vi "Changed Mode.vi"(8 "error in (no error)":errorcluster, 11 "Instrument in":refnum<class "Instrument.lvclass">) -> (0 "error out":errorcluster, 3 "Instrument out":refnum<class "Instrument.lvclass">)   [LabVIEW 2018, in "Instrument.lvclass"]
uses:
  Instrument.lvclass
  Instrument.lvclass/Instrument.ctl
  Device/Optics/Optics.lvclass/Optics.ctl
  Device/Optics/Opt_Selector/Opt_Selector.lvclass
  C:/Users/observer/Desktop/Sparc4GUI/SPARC4_GUI/Device/Optics/Optics.lvclass
  Device/Optics/Optics.lvclass
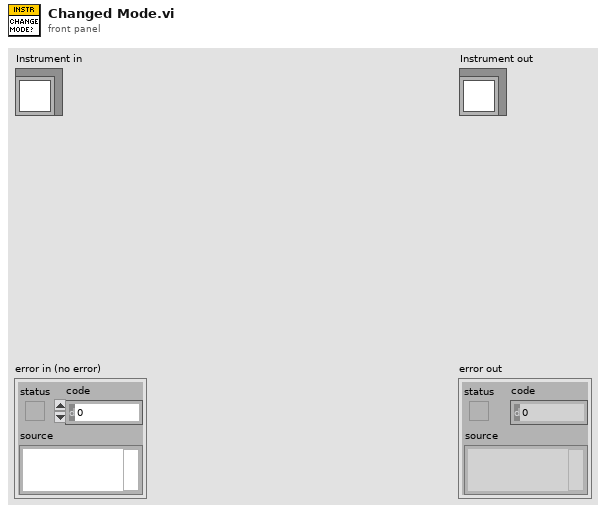
[diagram p1: front panel]
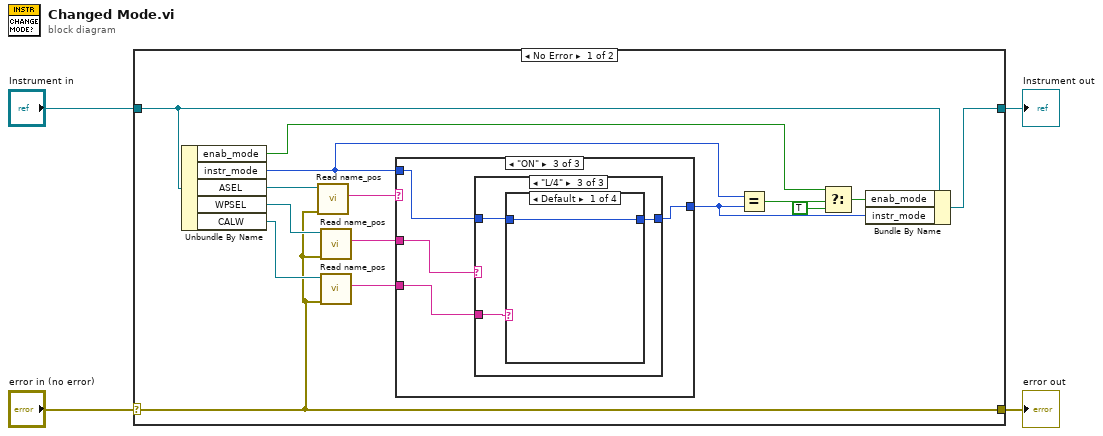
[diagram p0: block diagram]
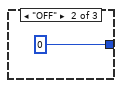
[diagram p3: hidden frame]
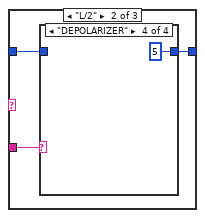
[diagram p5: hidden frame]
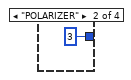
[diagram p7: hidden frame]
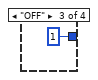
[diagram p8: hidden frame]
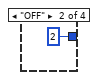
[diagram p9: hidden frame]
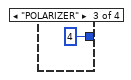
[diagram p10: hidden frame]
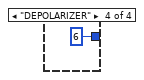
[diagram p11: hidden frame]
diagram:
  n1 = case shown="No Error" "error in (no error)" {
    selector: "error in (no error)" -> [w16 w42]
    tunnel: [w16 w42] -> w3
    tunnel: [w13 w41] -> w1
    tunnel: "Instrument in" -> [w14 w41]
    frame No Error {
      n2 = Unbundle By Name(w14) -> ("enab_mode"=w10:bool, "instr_mode"=w8:u32, "ASEL"=w19:refnum<class "Opt_Selector.lvclass">, "WPSEL"=w18:refnum<class "Opt_Selector.lvclass">, "CALW"=w17:refnum<class "Opt_Selector.lvclass">)
      n3 = call "Read name_pos.vi"("error in (no error)"=w16, "Optics in"=w19) -> ("name_pos"=w15:string)  [unwired: 7 in, 2 out]
      n4 = call "Read name_pos.vi"("error in (no error)"=w16, "Optics in"=w18) -> ("name_pos"=w6:string)  [unwired: 7 in, 2 out]
      n5 = call "Read name_pos.vi"("error in (no error)"=w16, "Optics in"=w17) -> ("name_pos"=w5:string)  [unwired: 7 in, 2 out]
      n6 = case shown="\"ON\"" w15 {
        tunnel: [w20 u32 0 w23] -> w7
        tunnel: w8 -> [w20 _ w24]
        tunnel: w6 -> [_ _ w25]
        tunnel: w5 -> [_ _ w22]
        frame Default {
        }
        frame "OFF" {
        }
        frame "ON" {
          n7 = case shown="\"L/4\"" w25 {
            tunnel: [w26 w27 w35] -> w23
            tunnel: w24 -> [w26 w28 w36]
            tunnel: w22 -> [_ w29 w34]
            frame Default {
            }
            frame "L/2" {
              n8 = case shown="\"DEPOLARIZER\"" w29 {
                tunnel: [w30 u32 3 ("instr_mode") u32 1 ("instr_mode") u32 5 ("instr_mode")] -> w27
                tunnel: w28 -> [w30 _ _ _]
                frame Default {
                }
                frame "POLARIZER" {
                }
                frame "OFF" {
                }
                frame "DEPOLARIZER" {
                }
              }
            }
            frame "L/4" {
              n9 = case shown="Default" w34 {
                tunnel: [w37 u32 2 ("instr_mode") u32 4 ("instr_mode") u32 6 ("instr_mode")] -> w35
                tunnel: w36 -> [w37 _ _ _]
                frame Default {
                }
                frame "OFF" {
                }
                frame "POLARIZER" {
                }
                frame "DEPOLARIZER" {
                }
              }
            }
          }
        }
      }
      n10 = Equal?(x=w8, y=w7) -> (x = y?=w11:bool)
      n11 = Select(t=w10, s=w11, f=TRUE) -> (s? t:f=w12:bool)
      n12 = Bundle By Name(cluster=w14, "enab_mode"=w12, "instr_mode"=w7) -> (w13:refnum<class "Instrument.lvclass">)
    }
    frame Error {
    }
  }
  "error out" <- w3
  "Instrument out" <- w1
